vi "Flywheel_Hardware_Globals.vi"() -> ()   [LabVIEW 2020]
panel:
  in  "Flywheel_Right":string="Flywheel_Right"
  in  "Flywheel_Left":string="Flywheel_Left"
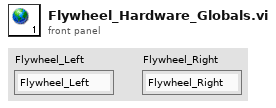
[diagram p1: front panel]
diagram:
